vi "Write_ProcessStartedMessage_VIRef.vi"(8 "error in (no error)":errorcluster, 10 "VI Refnum":refnum<vi>, 11 "ProcessStartedMessage in":refnum<class "ProcessStartedMessage.lvclass">) -> (0 "error out":errorcluster, 3 "ProcessStartedMessage out":refnum<class "ProcessStartedMessage.lvclass">)   [LabVIEW 2013, in "ProcessStartedMessage.lvclass"]
uses:
  ProcessStartedMessage.lvclass
  ProcessStartedMessage.lvclass/ProcessStartedMessage.ctl
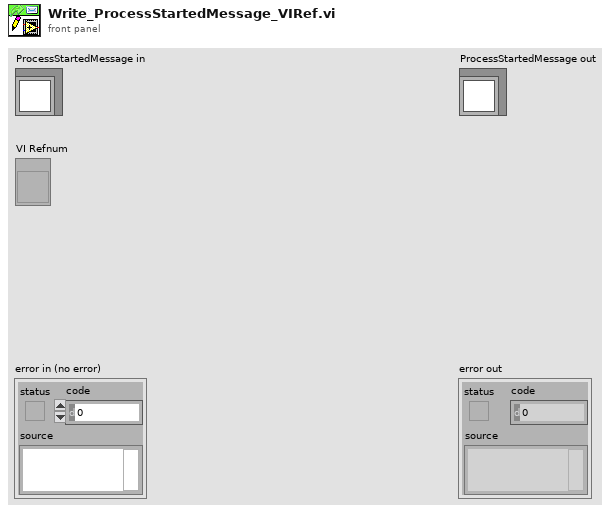
[diagram p1: front panel]
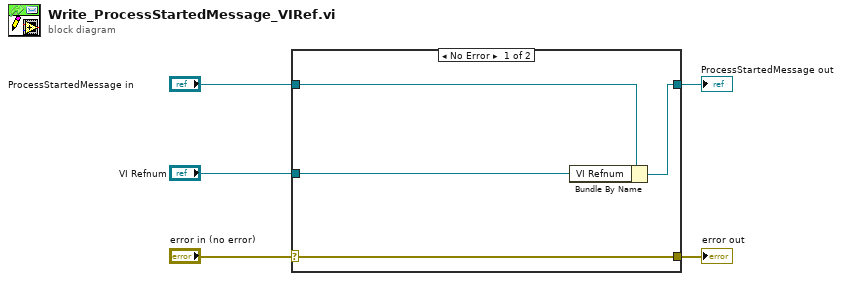
[diagram p0: block diagram]
diagram:
  n1 = case shown="No Error" "error in (no error)" {
    selector: "error in (no error)" -> [w9 w10]
    tunnel: [w9 w10] -> w4
    tunnel: [w7 w11] -> w2
    tunnel: "ProcessStartedMessage in" -> [w8 w11]
    tunnel: "VI Refnum" -> [w6 _]
    frame No Error {
      n2 = Bundle By Name(cluster=w8, "VI Refnum"=w6) -> (w7:refnum<class "ProcessStartedMessage.lvclass">)
    }
    frame Error {
    }
  }
  "error out" <- w4
  "ProcessStartedMessage out" <- w2
